vi "APS get feeder status.vi"(8 "error in (no error)":errorcluster caption="错误输入（无错误）", 9 "ErrCode":i32, 10 "State":i32, 11 "GroupId":i32) -> (0 "error out":errorcluster caption="错误输出", 1 "ErrCode out":i32, 2 "State out":i32, 3 "function return":i32)   [LabVIEW 2011, in "APS168.lvlib"]
doc: "I32 FNTYPE APS_get_feeder_status( I32 GroupId, I32 *State, I32 *ErrCode );"
uses:
  APS168.lvlib
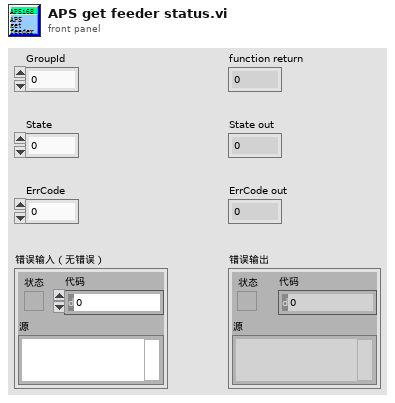
[diagram p1: front panel]
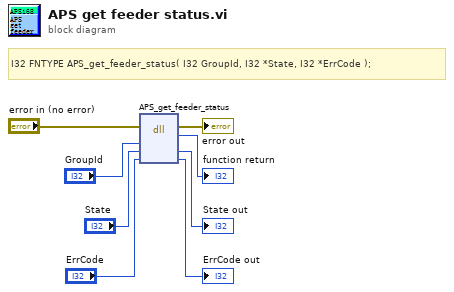
[diagram p0: block diagram]
diagram:
  # "I32 FNTYPE APS_get_feeder_status( I32 GroupId, I32 *State, I32 *ErrCode );"
  n1 = dll-call lib="PTH1Labs E软件ADLINK 204CAPS_1_7_1_LIB line 连续运动204APS168.*" fn="APS_get_feeder_status"(error in="error in (no error)", "GroupId"="GroupId", "State"="State", "ErrCode"="ErrCode") -> (error out=→"error out":errorcluster, →"function return":i32, "State"=→"State out":i32, "ErrCode"=→"ErrCode out":i32)  [unwired: 3 in, 1 out]
